vi "generatepockelscellarray for fast z.vi"(10 "interpolated pockels cell data":dbl[](array[numeric]), 11 "piezo control":dbl[](graph)) -> (3 "pockelscellarray":dbl[](array[numeric]))   [LabVIEW 2012]
uses:
  GFG/GFGnumericGet.vi
  GFG/GFG library.lvlib
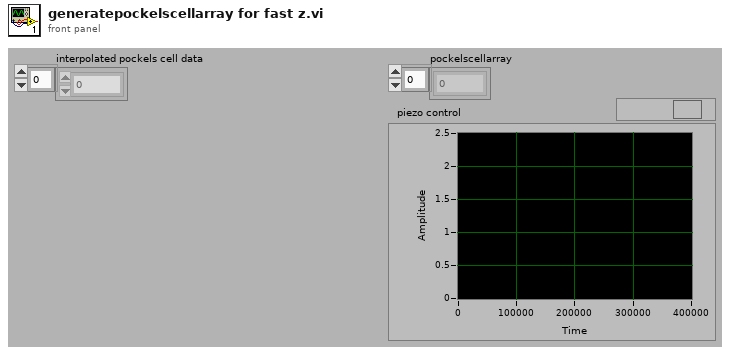
[diagram p1: front panel]
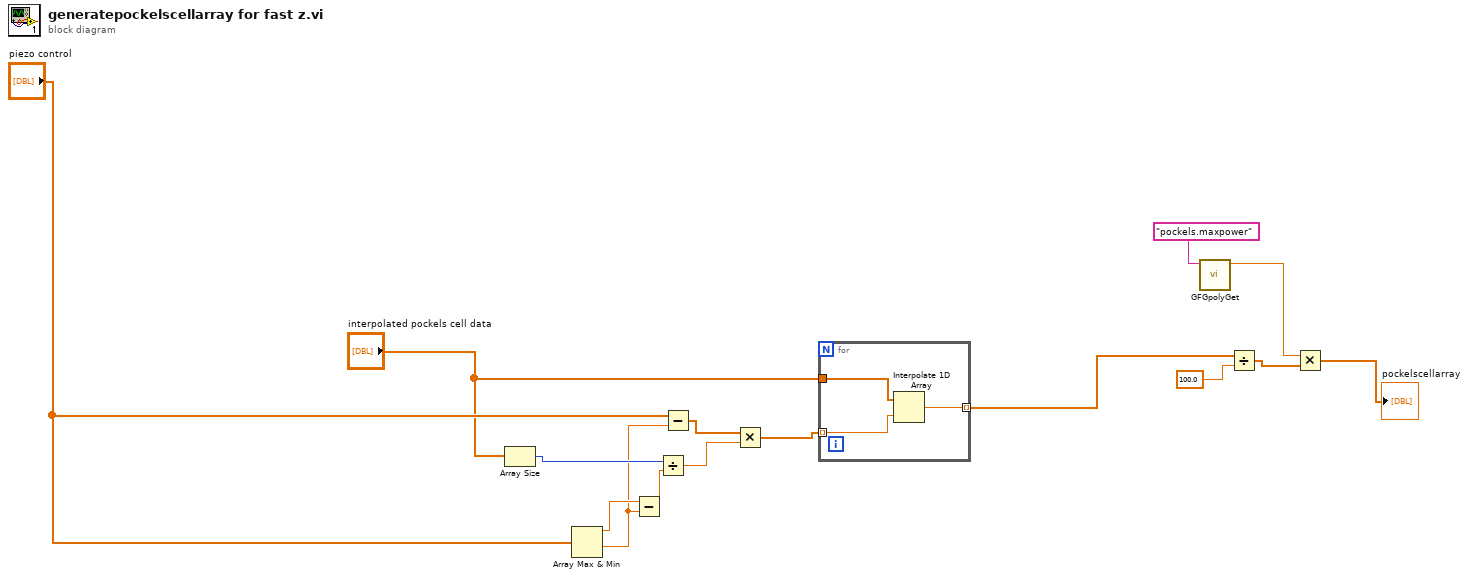
[diagram p0: block diagram]
diagram:
  n1 = Array Size(array="interpolated pockels cell data") -> (size(s)=w14:i32)
  n2 = Array Max & Min(array="piezo control") -> (max value=w12:dbl, min value=w9:dbl)  [unwired: 2 out]
  n3 = Subtract(x=w12, y=w9) -> (x-y=w11:dbl)
  n4 = Divide(x=w14, y=w11) -> (x/y=w13:dbl)
  n5 = Subtract(x="piezo control", y=w9) -> (x-y=w10:dbl[])
  n6 = Multiply(x=w10, y=w13) -> (x*y=w8:dbl[])
  n7 = for {
    tunnel: "interpolated pockels cell data" -> [w18]
    tunnel: [w17] -> w5 mode=indexing
    tunnel: w8 -> [w16] mode=indexing
    n8 = Interpolate 1D Array(1:w16, 2:w18) -> (0:w17:dbl)
  }
  n9 = call-poly "GFGpolyGet.vi"("Variable Name in"="pockels.maxpower") -> ("Numeric"=w1:dbl)  [unwired: 9 in, 1 out]
  n10 = Divide(x=w5, y=100.0 ("x")) -> (x/y=w6:dbl[])
  n11 = Multiply(x=w1, y=w6) -> (x*y=→"pockelscellarray":dbl[])
